vi "GetSingleCalibrationMethod.vi"(8 "error in (no error)":errorcluster, 10 "ID":string, 11 "ByteGSWebAPI-V0 in":refnum<class "ByteGSWebAPI-V0.lvclass">) -> (0 "error out":errorcluster, 2 "SingleCalibrationMethod":T1, 3 "ByteGSWebAPI-V0 out":refnum<class "ByteGSWebAPI-V0.lvclass">)   [LabVIEW 2019, in "ByteGSWebAPI-V0.lvclass"]
doc: "Richiesta di GET di calibration method identificato da un ID in ingresso"
uses:
  ByteGSWebAPI-V0.lvclass
  Cntrls/SingleCalibrationMethod.ctl
  54c15d21-1fd3-4ea8-80e2-c69b0da6434b.vi
  <vilib>/JDP Science/JSONtext/JSON text to Variant.vi
  <vilib>/JDP Science/JSONtext/LVClass Serializer/JSONtext LVClass Serializer.lvclass
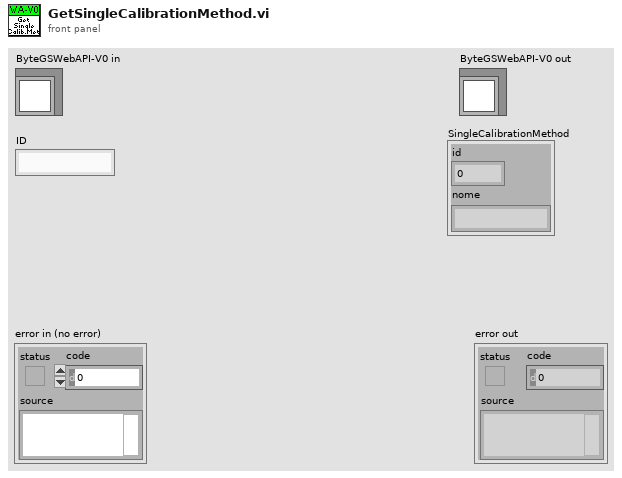
[diagram p1: front panel]
types:
  T1 = typedef "ByteGSWebAPI-V0.lvclass/SingleCalibrationMethod.ctl" = cluster{"id":i32, "nome":string}
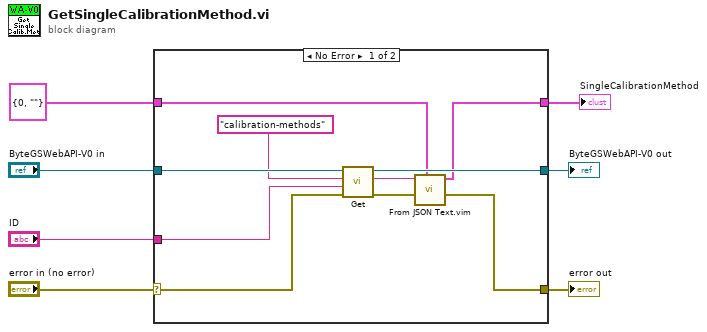
[diagram p0: block diagram]
diagram:
  n1 = case shown="No Error" "error in (no error)" {
    selector: "error in (no error)" -> [w13 w19]
    tunnel: [w10 w19] -> w6
    tunnel: [w15 w18] -> w4
    tunnel: "ByteGSWebAPI-V0 in" -> [w16 w18]
    tunnel: "ID" -> [w12 _]
    tunnel: T1 {"id"=0, "nome"=""} ("SingleCalibrationMethod") -> [w9 w17]
    tunnel: [w8 w17] -> w1
    frame No Error {
      n2 = call "Get.vi"("error in (no error)"=w13, "Parameter"=w12, "Request"="calibration-methods" ("Parameter"), "ByteGSWebAPI-V0 in"=w16) -> ("error out"=w10:errorcluster, "body"=w11:string, "ByteGSWebAPI-V0 out"=w15:refnum<class "ByteGSWebAPI-V0.lvclass">)  [unwired: 4 in, 1 out]
      n3 = call "From JSON Text.vim"("Data Type and Default Value"=w9, "error in (no error)"=w10, "JSON"=w11) -> ("Data out"=w8:T1)  [unwired: 7 in, 1 out]
    }
    frame Error {
    }
  }
  "error out" <- w6
  "ByteGSWebAPI-V0 out" <- w4
  "SingleCalibrationMethod" <- w1
